vi "Add_TCPRef_IP_port.vi"(6 "TCP Ref":refnum<k5>, 8 "error in":errorcluster caption="错误输入", 9 "port":u16, 11 "IP":string) -> (0 "error out":errorcluster caption="错误输出")   [LabVIEW 2015]
uses:
  Global/SeverGlobal.vi
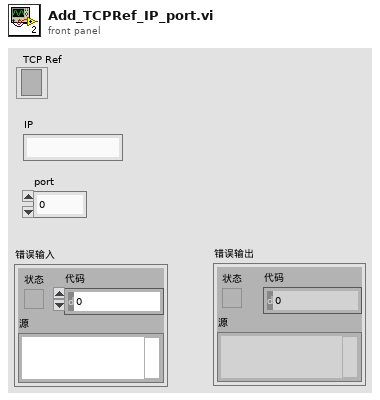
[diagram p1: front panel]
types:
  T1 = cluster{"TCP Ref":refnum<k5>, "Broadcast":refnum<k5>, "TF":refnum<k5>, "IP":string, "port":u16, "userName":string, "passWord":string, "authority":string}
  T2 = cluster{"TCP Ref":refnum<k5>, "Broadcast":refnum<k5>, "TF Ref":refnum<k5>, "IP":string, "port":u16, "userName":string, "passWord":string, "authority":string}[]
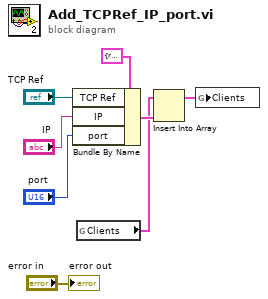
[diagram p0: block diagram]
diagram:
  n1 = Bundle By Name(cluster=T1 {"TCP Ref"=refnum, "Broadcast"=refnum, "TF"=refnum, "IP"="", "port"=0, "userName"="", "passWord"="", "authority"=""} ("Client"), "TCP Ref"="TCP Ref", "IP"="IP", "port"="port") -> (w5:T1)
  n2 = global read "SeverGlobal.vi" "Clients"() -> (w4:T2)
  n3 = Insert Into Array(array=w4, new element=w5) -> (w3:T2)  [unwired: 1 in]
  n4 = global write "SeverGlobal.vi" "Clients"(w3) -> ()
  "error out" <- "error in"
